vi "COM Port selector español.vi"() -> (2 "Cancelled?":bool, 3 "VISA Refnum out":refnum<visa-resource-name>)   [LabVIEW 2025, in "Control de MaP.lvlib"]
uses:
  Control de MaP.lvlib
panel:
  in  "OK Button":bool
  in  "Puerto COM":refnum<visa-resource-name>="COM4"
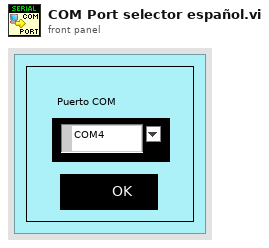
[diagram p1: front panel]
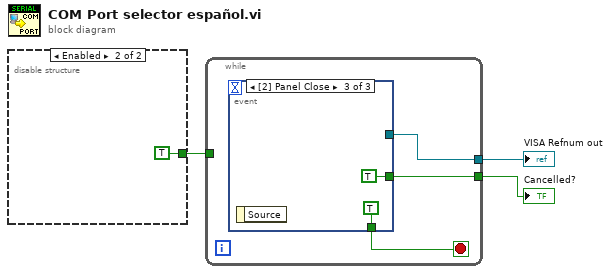
[diagram p0: block diagram]
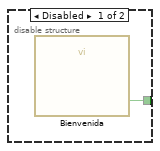
[diagram p2: hidden frame]
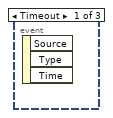
[diagram p3: hidden frame]
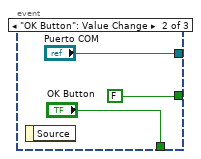
[diagram p4: hidden frame]
diagram:
  n1 = disable-structure shown="Enabled" {
    disable-tunnel: [w4 TRUE ("OK")] -> w2
    frame Disabled {
      n2 = call "Bienvenida"() -> ("OK"=w4:bool)  [unwired: 18 in, 1 out]
    }
    frame Enabled {
    }
  }
  n3 = while {
    tunnel: [w7] -> w3
    tunnel: w2 -> [_]
    tunnel: [w6] -> w1
    stop <- w8 stop-if-true
    n4 = event shown="[2] Panel Close" {
      selector: _ -> [_ _ _]
      dyn-events: _ -> [_ _ _]
      timeout: _ -> [_ _ _]
      tunnel: [_ "OK Button" TRUE ("OK Button")] -> w8
      tunnel: [_ "Puerto COM" _] -> w7
      tunnel: [_ FALSE TRUE] -> w6
      event Timeout {
        n5 = event-data() -> ()  [unwired: 1 in, 3 out]
      }
      event "OK Button": Value Change {
        n6 = event-data() -> ()  [unwired: 1 in, 1 out]
      }
      event Panel Close {
        n7 = event-data() -> ()  [unwired: 1 in, 1 out]
      }
    }
  }
  "VISA Refnum out" <- w3
  "Cancelled?" <- w1
